vi "EditParabola.vi"() -> ()   [LabVIEW 2020, in "Curve Editor.lvlib"]
uses:
  Curve Editor.lvlib
  Key Value/Key Value.lvlib
panel:
  in  "偏移量c":dbl format="%.2f"
  in  "平移量b":dbl format="%.2f"
  in  "系数a":dbl format="%.2f"
  in  "时间[S]":dbl format="%.2f"
  in  "Tree引用句柄":refnum<vi>
  in  "索引":i32
  in  "取消按钮":bool
  in  "确定按钮":bool
  # "f(x)=a(x+b)^2+c"
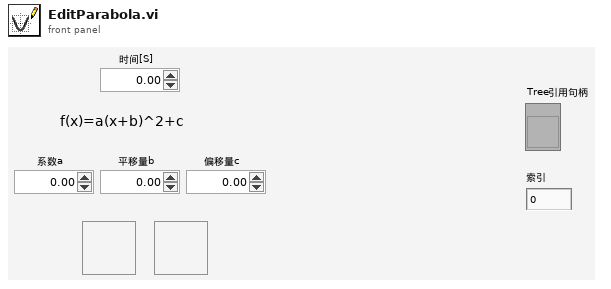
[diagram p1: front panel]
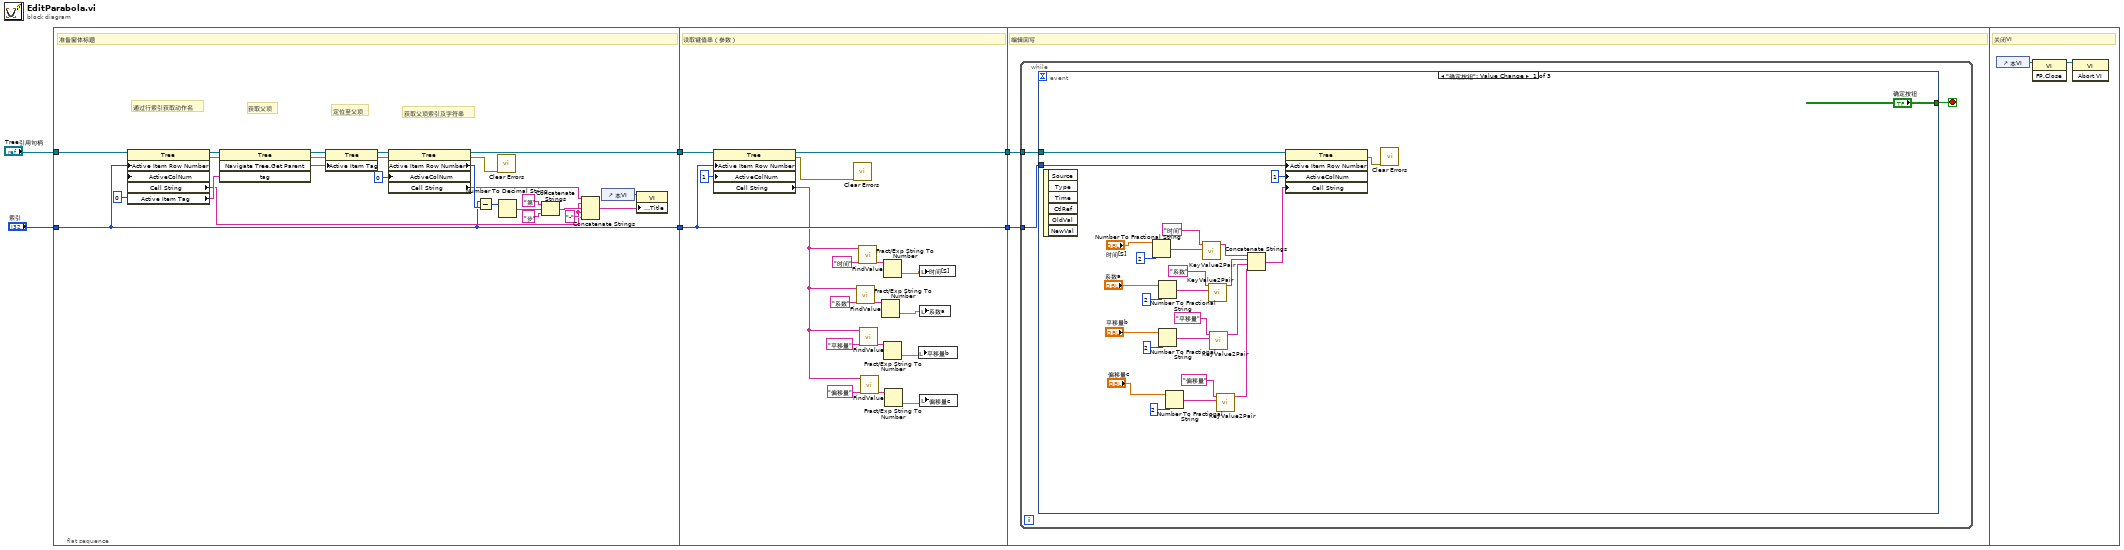
[diagram p0: block diagram]
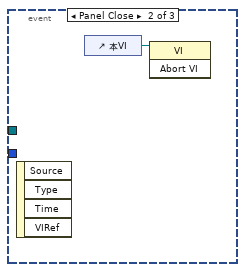
[diagram p2: hidden frame]
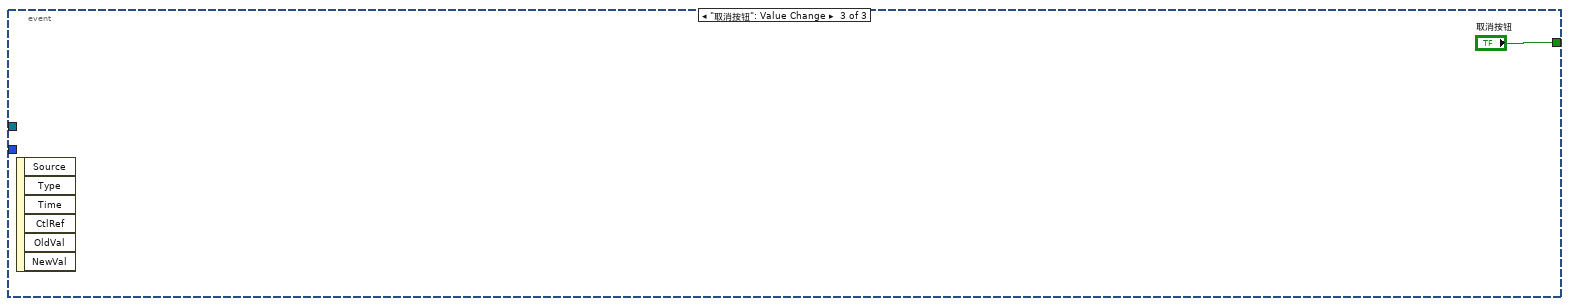
[diagram p3: hidden frame]
diagram:
  n1 = flat-sequence {
    tunnel: [w13] -> w6
    tunnel: [w12] -> w4
    tunnel: "Tree引用句柄" -> [w14]
    tunnel: "索引" -> [w13]
    tunnel: w6 -> [w47]
    tunnel: [w47] -> w5
    tunnel: w4 -> [w48]
    tunnel: [w46] -> w3
    tunnel: w5 -> [w51]
    tunnel: w3 -> [w50]
    frame #0 {
      w16 = "-" ("字符串")
      # "获取父项索引及字符串"
      # "定位至父项"
      # "获取父项"
      # "通过行索引获取动作名"
      # "准备窗体标题"
      n2 = property class="Tree"(reference=w14, "Active Item Row Number"=w13, "ActiveColNum"=0 ("活动单元格:活动列数")) -> (reference out=w11:refnum<vi>, error out=w10:errorcluster, "Cell String"=w15:string, "Active Item Tag"=w28:string)  [unwired: 1 in]
      n3 = invoke class="Tree" method="Navigate Tree.Get Parent"(reference=w11, error in=w10, "tag"=w28) -> (reference out=w23:refnum<vi>, error out=w9:errorcluster, "Navigate Tree:Get Parent"=w24:string)  [unwired: 1 in, 1 out]
      n4 = property class="Tree"(reference=w23, error in=w9, "Active Item Tag"=w24) -> (reference out=w22:refnum<vi>, error out=w8:errorcluster)
      n5 = property class="Tree"(reference=w22, error in=w8, "ActiveColNum"=0 ("活动单元格:活动列数")) -> (reference out=w12:refnum<vi>, error out=w7:errorcluster, "Active Item Row Number"=w26:i32, "Cell String"=w25:string)
      n6 = Subtract(x=w13, y=w26) -> (x-y=w21:i32)
      n7 = call <vilib>:"Clear Errors.vi"("error in (no error)"=w7) -> ()  [unwired: 5 in, 2 out]
      n8 = Number To Decimal String(number=w21) -> (decimal integer string=w19:string)  [unwired: 1 in]
      n9 = Concatenate Strings("第", w19, "步") -> (w17:string)
      n10 = Concatenate Strings(w25, w16, w17, w16, w15) -> (w29:string)
      n11 = control-ref of="本VI"() -> (w31:refnum<vi>)
      n12 = property class="VI"(reference=w31, "Front Panel.Title"=w29) -> ()  [unwired: 1 in, 2 out]
    }
    frame #1 {
      # "读取键值串（参数）"
      n13 = property class="Tree"(reference=w48, "Active Item Row Number"=w47, "ActiveColNum"=1 ("活动单元格:活动列数")) -> (reference out=w46:refnum<vi>, error out=w32:errorcluster, "Cell String"=w33:string)  [unwired: 1 in]
      n14 = call <vilib>:"Clear Errors.vi"("error in (no error)"=w32) -> ()  [unwired: 5 in, 2 out]
      n15 = call "FindValue.vi"("键"="系数", "键值串"=w33) -> ("值"=w41:string)  [unwired: 8 in, 1 out]
      n16 = call "FindValue.vi"("键"="时间", "键值串"=w33) -> ("值"=w44:string)  [unwired: 8 in, 1 out]
      n17 = call "FindValue.vi"("键"="平移量", "键值串"=w33) -> ("值"=w38:string)  [unwired: 8 in, 1 out]
      n18 = call "FindValue.vi"("键"="偏移量", "键值串"=w33) -> ("值"=w35:string)  [unwired: 8 in, 1 out]
      n19 = Fract/Exp String To Number(string=w41) -> (number=w42:dbl)  [unwired: 3 in, 1 out]
      n20 = Fract/Exp String To Number(string=w44) -> (number=w43:dbl)  [unwired: 3 in, 1 out]
      n21 = Fract/Exp String To Number(string=w38) -> (number=w37:dbl)  [unwired: 3 in, 1 out]
      n22 = Fract/Exp String To Number(string=w35) -> (number=w34:dbl)  [unwired: 3 in, 1 out]
      n23 = local write "平移量b"(w37) -> ()
      n24 = local write "时间[S]"(w43) -> ()
      n25 = local write "系数a"(w42) -> ()
      n26 = local write "偏移量c"(w34) -> ()
    }
    frame #2 {
      # "编辑回写"
      n27 = while {
        tunnel: w51 -> [w53]
        tunnel: w50 -> [w52]
        stop <- w54 stop-if-true
        n28 = event shown="[0] \"确定按钮\": Value Change" {
          selector: _ -> [_ _ _]
          dyn-events: _ -> [_ _ _]
          timeout: _ -> [_ _ _]
          tunnel: ["确定按钮" _ "取消按钮"] -> w54
          tunnel: w53 -> [w79 _ _]
          tunnel: w52 -> [w78 _ _]
          event "确定按钮": Value Change {
            n29 = event-data() -> ()  [unwired: 1 in, 6 out]
            n30 = Number To Fractional String(number="时间[S]", precision (6)=i16 2 ("精度(6)")) -> (F-format string=w75:string)  [unwired: 2 in]
            n31 = Number To Fractional String(number="系数a", precision (6)=i16 2 ("精度(6)")) -> (F-format string=w72:string)  [unwired: 2 in]
            n32 = Number To Fractional String(number="平移量b", precision (6)=i16 2 ("精度(6)")) -> (F-format string=w69:string)  [unwired: 2 in]
            n33 = Number To Fractional String(number="偏移量c", precision (6)=i16 2 ("精度(6)")) -> (F-format string=w59:string)  [unwired: 2 in]
            n34 = call "KeyValue2Pair.vi"("值"=w75, "键"="时间") -> ("键值对"=w64:string)  [unwired: 9 in]
            n35 = call "KeyValue2Pair.vi"("值"=w72, "键"="系数") -> ("键值对"=w63:string)  [unwired: 9 in]
            n36 = call "KeyValue2Pair.vi"("值"=w69, "键"="平移量") -> ("键值对"=w62:string)  [unwired: 9 in]
            n37 = call "KeyValue2Pair.vi"("值"=w59, "键"="偏移量") -> ("键值对"=w56:string)  [unwired: 9 in]
            n38 = Concatenate Strings(w64, w63, w62, w56) -> (w61:string)
            n39 = property class="Tree"(reference=w78, "Active Item Row Number"=w79, "ActiveColNum"=1 ("活动单元格:活动列数"), "Cell String"=w61) -> (error out=w55:errorcluster)  [unwired: 1 in, 1 out]
            n40 = call <vilib>:"Clear Errors.vi"("error in (no error)"=w55) -> ()  [unwired: 5 in, 2 out]
          }
          event Panel Close {
            n41 = event-data() -> ()  [unwired: 1 in, 4 out]
            n42 = control-ref of="本VI"() -> (w81:refnum<vi>)
            n43 = invoke class="VI" method="Abort VI"(reference=w81) -> ()  [unwired: 2 in, 3 out]
          }
          event "取消按钮": Value Change {
            n44 = event-data() -> ()  [unwired: 1 in, 6 out]
          }
        }
      }
    }
    frame #3 {
      # "关闭VI"
      n45 = control-ref of="本VI"() -> (w84:refnum<vi>)
      n46 = invoke class="VI" method="FP.Close"(reference=w84) -> (reference out=w83:refnum<vi>)  [unwired: 2 in, 2 out]
      n47 = invoke class="VI" method="Abort VI"(reference=w83) -> ()  [unwired: 2 in, 3 out]
    }
  }
